vi "plotting chart graph.vi"() -> ()   [LabVIEW 2012]
panel:
  out "Waveform Graph":dbl[](graph)
  out "Waveform Chart 3":dbl(graph)
  out "Waveform Chart 2":dbl(graph)
  out "Waveform Chart":dbl(graph)
  in  "stop":bool
  # "SCOPE"
  # "STRIP"
  # "SWEEP"
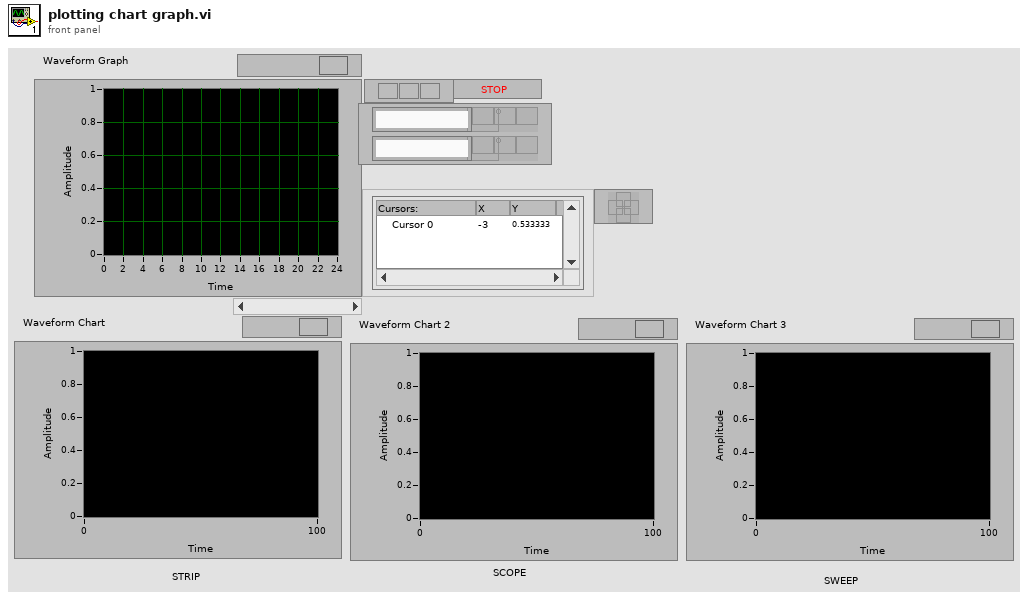
[diagram p1: front panel]
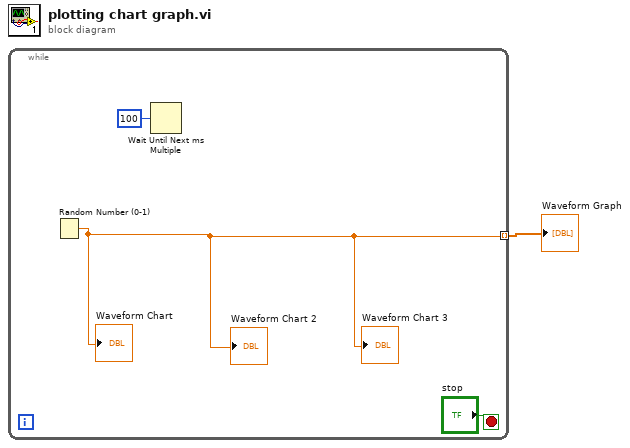
[diagram p0: block diagram]
diagram:
  n1 = while {
    tunnel: [w3] -> w1 mode=indexing
    stop <- "stop" stop-if-true
    n2 = Random Number (0-1)() -> (number: 0 to 1=w3:dbl)
    "Waveform Chart" <- w3
    "Waveform Chart 2" <- w3
    "Waveform Chart 3" <- w3
    n3 = Wait Until Next ms Multiple(millisecond multiple=u32 100) -> ()  [unwired: 1 out]
  }
  "Waveform Graph" <- w1
